vi "Write system-defined metadata.vi"(8 "error in (no error)":errorcluster, 10 "Get Object Result Parameters":T1, 11 "Object in":refnum<class "Object.lvclass">) -> (0 "error out":errorcluster, 3 "Object out":refnum<class "Object.lvclass">)   [LabVIEW 2015, in "NI_AWS_S3.lvlib" / "Object.lvclass"]
uses:
  Object.lvclass
  GET Object Result Parameters.ctl
  Object.lvclass/Object.ctl
  NI_AWS_S3.lvlib
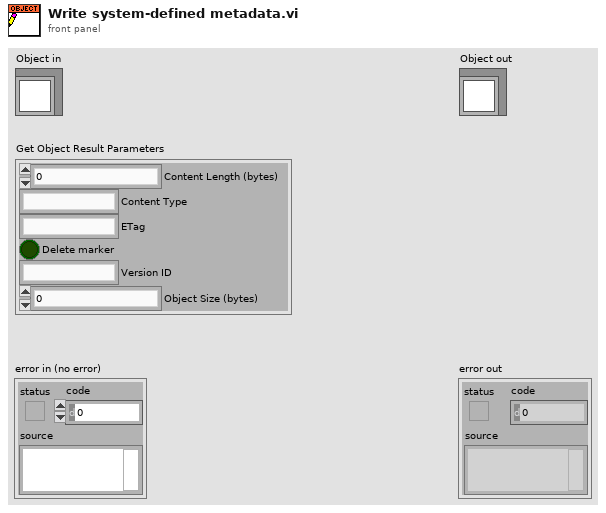
[diagram p1: front panel]
types:
  T1 = typedef "NI_AWS_S3.lvlib/GET Object Result Parameters.ctl" = cluster{"Content Length (bytes)":u64, "Content Type":string, "ETag":string, "Delete marker":bool, "Version ID":string, "Object Size (bytes)":u64}
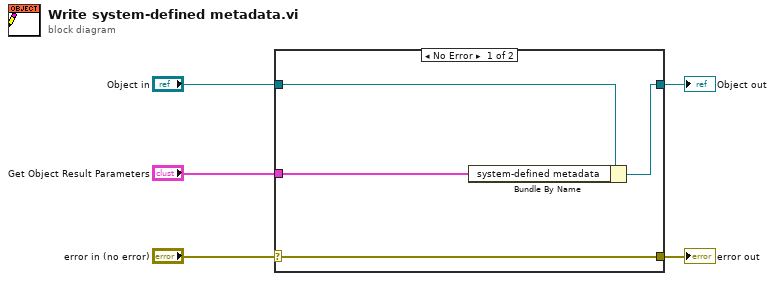
[diagram p0: block diagram]
diagram:
  n1 = case shown="No Error" "error in (no error)" {
    selector: "error in (no error)" -> [w9 w10]
    tunnel: [w9 w10] -> w4
    tunnel: [w7 w11] -> w2
    tunnel: "Object in" -> [w8 w11]
    tunnel: "Get Object Result Parameters" -> [w6 _]
    frame No Error {
      n2 = Bundle By Name(cluster=w8, "system-defined metadata"=w6) -> (w7:refnum<class "Object.lvclass">)
    }
    frame Error {
    }
  }
  "error out" <- w4
  "Object out" <- w2
